vi "Add Message.vi"(0 "PainOutputTerminal in":refnum<class "SystemLinkOutputTerminal.lvclass">, 5 "Line Number":i64, 7 "Message":string, 11 "error in (no error)":errorcluster) -> (4 "PainOutputTerminal out":refnum<class "SystemLinkOutputTerminal.lvclass">, 15 "error out":errorcluster)   [LabVIEW 2016, in "SystemLinkOutputTerminal.lvclass"]
uses:
  SystemLinkOutputTerminal.lvclass
  Plain OT/PainOutputTerminal.lvclass
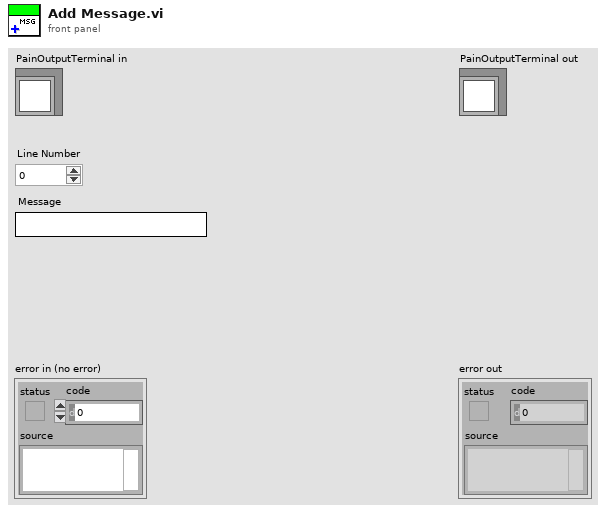
[diagram p1: front panel]
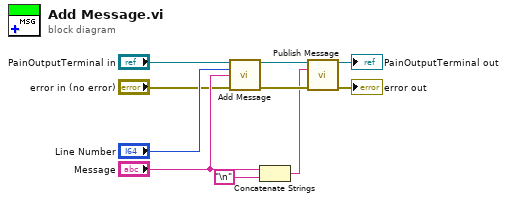
[diagram p0: block diagram]
diagram:
  n1 = call-parent "Add Message.vi"("PainOutputTerminal in"="PainOutputTerminal in", "Line Number"="Line Number", "Message"="Message", "error in (no error)"="error in (no error)") -> ("PainOutputTerminal out"=w4:refnum<class "SystemLinkOutputTerminal.lvclass">, "error out"=w5:errorcluster)  [unwired: 10 in]
  n2 = Concatenate Strings("Message", "\n" ("string")) -> (w1:string)
  n3 = call "Publish Message.vi"("SystemLinkOutputTerminal in"=w4, "Publish Message"=w1, "error in (no error)"=w5) -> ("SystemLinkOutputTerminal out"=→"PainOutputTerminal out":refnum<class "SystemLinkOutputTerminal.lvclass">, "error out"=→"error out":errorcluster)  [unwired: 11 in]
